vi "Timestamp to SQL Time.vi"(9 "Time Datatype":T1, 11 "Timestamp":timestamp) -> (3 "date/time string":string)   [LabVIEW 2019, in "LV-Data.PGSQL.lvclass"]
uses:
  LV-Data.PGSQL.lvclass
  Typedefs/Time.Datatype--enum.ctl
  <vilib>/LabVIEW Open Source Project/Epoch Date & Time/formatter.iso8601/Seconds Units -- enum.ctl
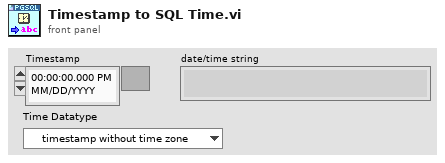
[diagram p1: front panel]
types:
  T1 = typedef "LV-Data.PGSQL.lvclass/Time.Datatype--enum.ctl" = enum16{"timestamp without time zone", "timestamp with time zone"}
  T2 = typedef "Seconds Units -- enum.ctl" = enum16{"second", "millisecond", "microsecond", "nanosecond"}
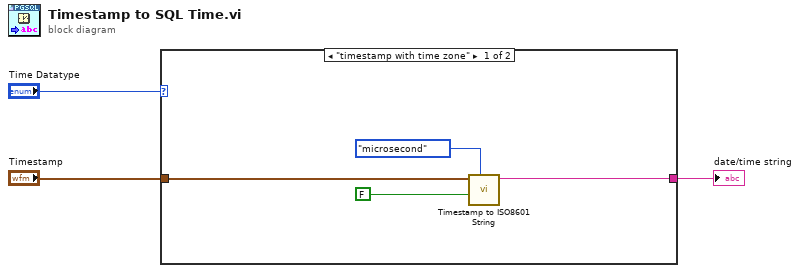
[diagram p0: block diagram]
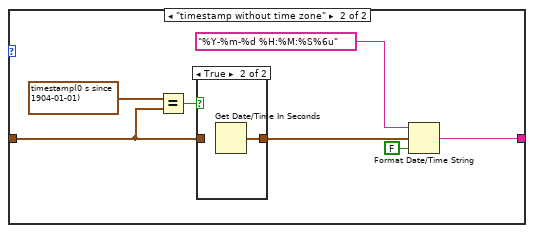
[diagram p2: hidden frame]
diagram:
  n1 = case shown="\"timestamp with time zone\"" "Time Datatype" {
    tunnel: [w5 w14] -> w3
    tunnel: "Timestamp" -> [w7 w11]
    frame "timestamp with time zone" {
      n2 = call <vilib>:"Timestamp to ISO8601 String.vi"("Unit (ms)"=Seconds_Units_--_enum."microsecond", "UTC? (F)"=FALSE, "Timestamp (now)"=w7) -> ("ISO8601 String"=w5:string)  [unwired: 8 in]
    }
    frame "timestamp without time zone" {
      n3 = Equal?(x=timestamp(0 s since 1904-01-01), y=w11) -> (x = y?=w13:bool)
      n4 = case shown="True" w13 {
        tunnel: [w15 w16] -> w10
        tunnel: w11 -> [w15 _]
        frame False {
        }
        frame True {
          n5 = Get Date/Time In Seconds() -> (seconds since 1Jan1904=w16:timestamp)
        }
      }
      n6 = Format Date/Time String(time format string (%c)="%Y-%m-%d %H:%M:%S%6u", seconds (now)=w10, UTC format=FALSE) -> (date/time string=w14:string)
    }
  }
  "date/time string" <- w3
